vi "voltageCheck.vi"() -> ()   [LabVIEW 2021]
panel:
  out "Color Box":u32(colorbox)
  in  "Voltage control  2":dbl(knob) scale=0.0..5.0
  out "?":string
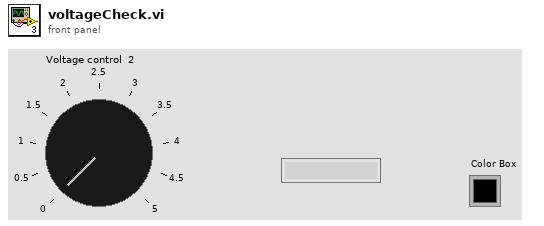
[diagram p1: front panel]
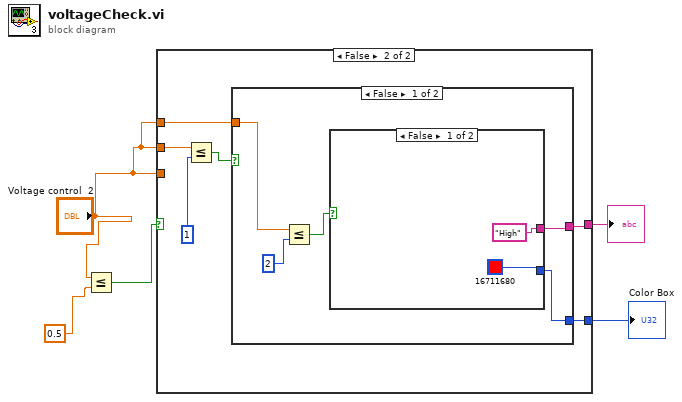
[diagram p0: block diagram]
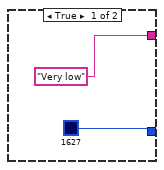
[diagram p2: hidden frame]
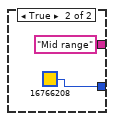
[diagram p3: hidden frame]
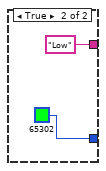
[diagram p4: hidden frame]
diagram:
  n1 = Less Or Equal?(x="Voltage control  2", y=0.5) -> (x <= y?=w4:bool)
  n2 = case shown="False" w4 {
    tunnel: ["Very low" w10] -> w2
    tunnel: "Voltage control  2" -> [_ _]
    tunnel: "Voltage control  2" -> [_ w12]
    tunnel: "Voltage control  2" -> [_ w9]
    tunnel: [u32 1627 ("Color Box 2") w8] -> w1
    frame True {
    }
    frame False {
      n3 = Less Or Equal?(x=w12, y=1) -> (x <= y?=w13:bool)
      n4 = case shown="False" w13 {
        tunnel: [w15 "Low"] -> w10
        tunnel: w9 -> [w16 _]
        tunnel: [w14 u32 65302 ("Color Box 2")] -> w8
        frame False {
          n5 = Less Or Equal?(x=w16, y=2) -> (x <= y?=w18:bool)
          n6 = case shown="False" w18 {
            tunnel: ["High" "Mid range"] -> w15
            tunnel: [u32 16711680 ("Color Box 2") u32 16766208 ("Color Box 2")] -> w14
            frame False {
            }
            frame True {
            }
          }
        }
        frame True {
        }
      }
    }
  }
  "?" <- w2
  "Color Box" <- w1
